vi "create odor and manifold configuration (sub-vi).vi"(7 "default directory (none)":path, 8 "error in (no error)":errorcluster, 10 "use initial config? (F)":bool, 11 "initial odor and manifold config (none)":T1) -> (0 "error out":errorcluster, 2 "operation failed?":bool, 3 "odor and manifold config out":T1)   [LabVIEW 2021]
uses:
  type-defs/odor description array (type def).ctl
  type-defs/odor info cluster (type def).ctl
  type-defs/odor selection (type def).ctl
  type-defs/odor color (type def).ctl
  type-defs/manifold configuration cluster array (type def).ctl
  type-defs/manifold configuration cluster (type def).ctl
  type-defs/manifold selection.ctl
  type-defs/single port single odor cluster.ctl
  type-defs/port number (type def).ctl
  type-defs/odor and manifold config UI states (type def).ctl
  type-defs/odor and manifold config cluster (type def).ctl
  <vilib>/Utility/error.llb/DialogType.ctl
  global-variables/global variables.vi
  <vilib>/Utility/error.llb/Error Cluster From Error Code.vi
  <vilib>/ErrorRing/Error Ring.xnode
panel:
  out "value error source":string
  in  "load config":bool
  in  "save config":bool
  in  "confirm button":bool
  out "state":T11
  out "cycle number":i32
  in  "odor config":T9 caption="Configure Odor Channels"
  in  "manifold config":T2 caption="Configure Manifold Ports"
  in  "cancel button":bool
  # "File"
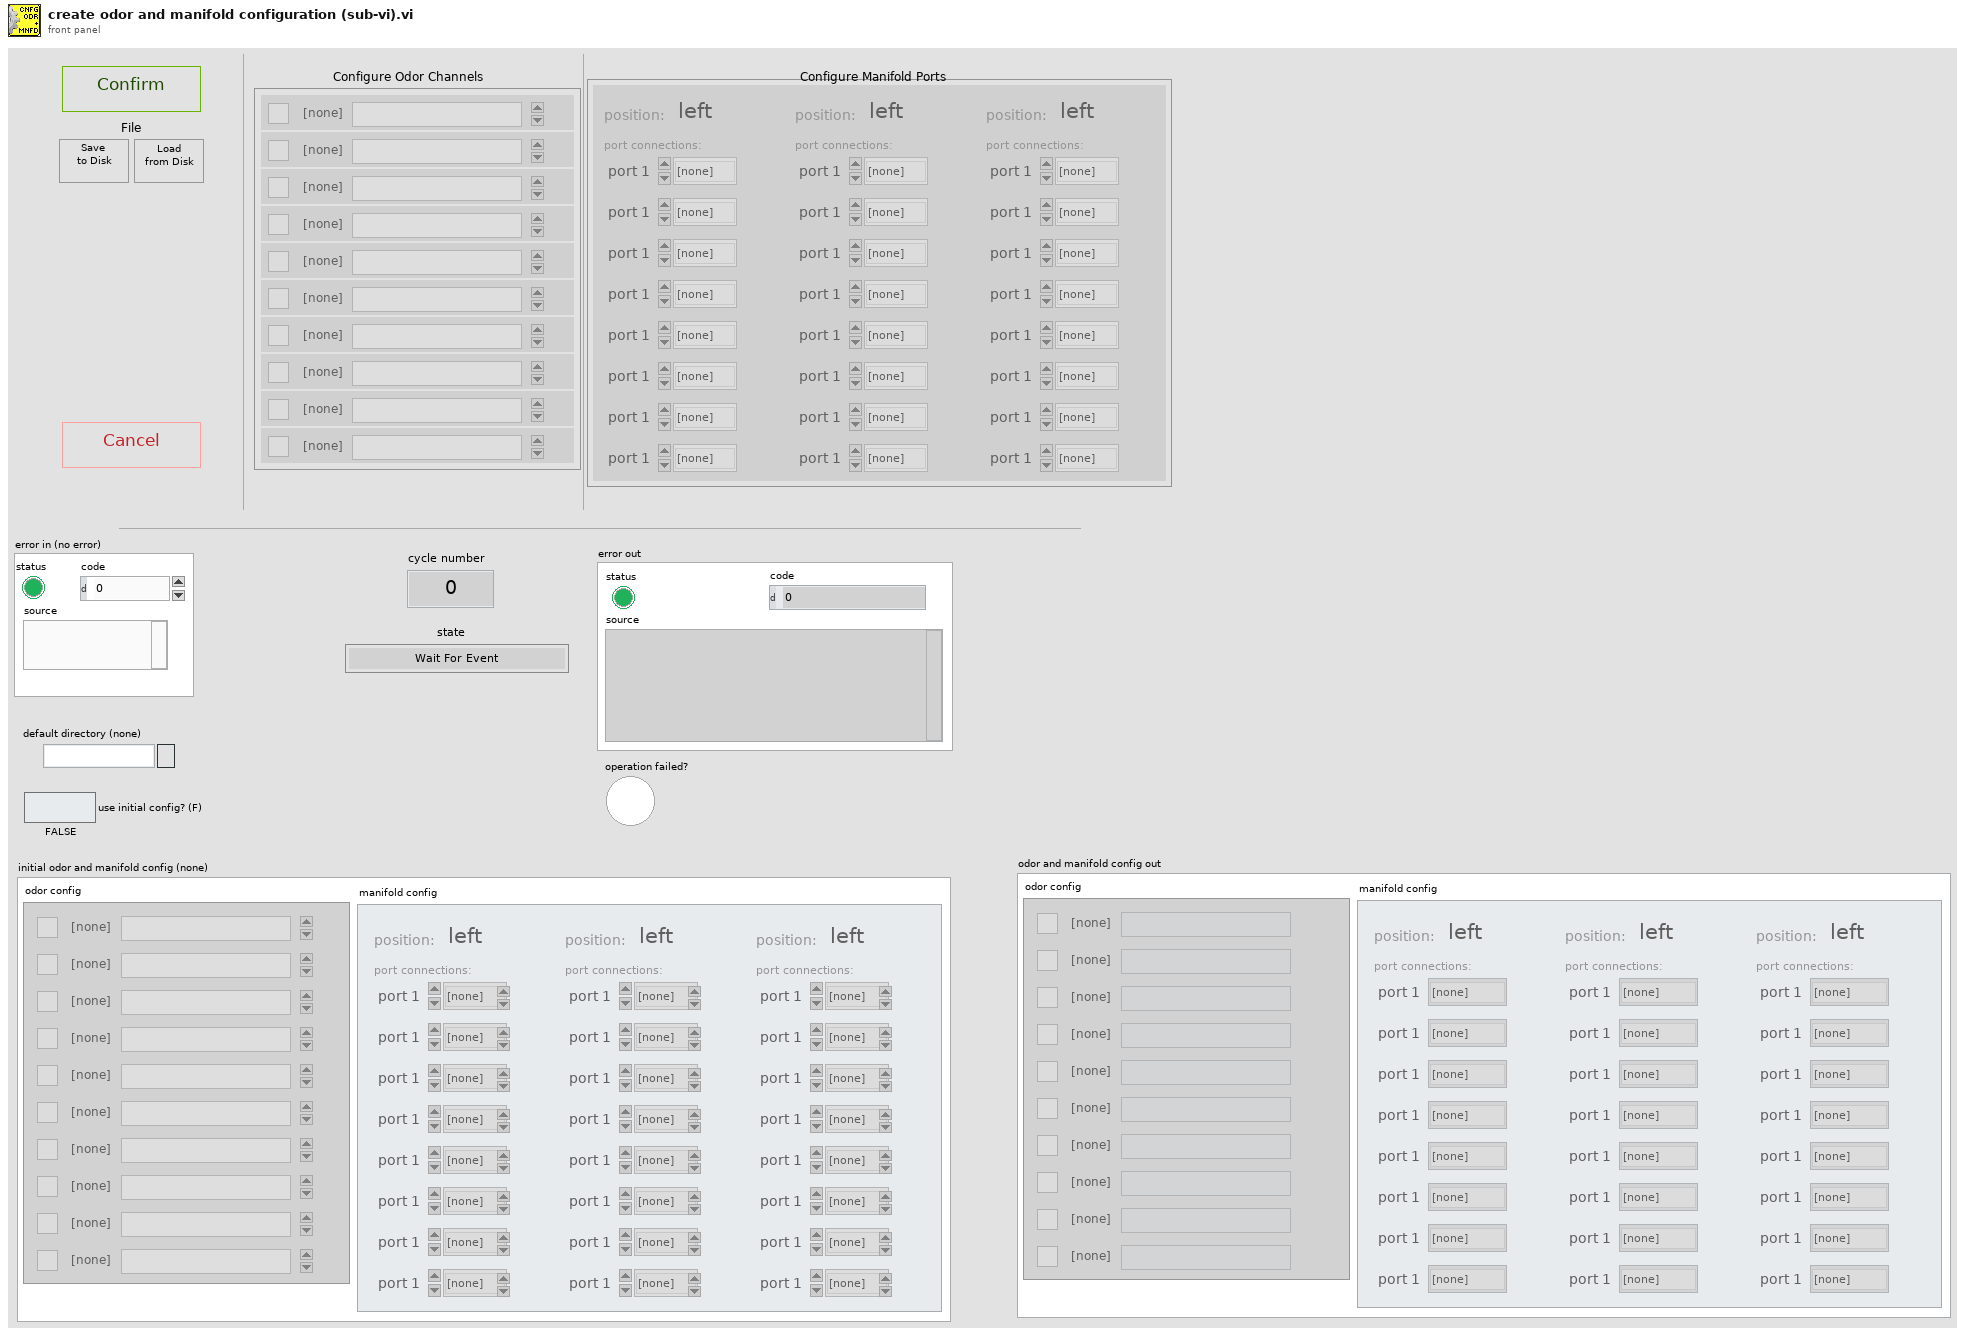
[diagram p1: front panel]
types:
  T1 = typedef "odor and manifold config cluster (type def).ctl" = cluster{"manifold config":T2, "odor config":T9}
  T2 = typedef "manifold configuration cluster array (type def).ctl" = T3[]
  T3 = typedef "manifold configuration cluster (type def).ctl" = cluster{"position:":T4, "port connections:":T5[]}
  T4 = typedef "manifold selection.ctl" = enum16{"left", "middle", "right"}
  T5 = typedef "single port single odor cluster.ctl" = cluster{"port number":T6, "connected odor":T7, "error":bool, "odor color":T8}
  T6 = typedef "port number (type def).ctl" = enum16{"port 1", "port 2", "port 3", "port 4", "port 5", "port 6", "port 7", "port 8"}
  T7 = typedef "odor selection (type def).ctl" = enum16{"[none]", "odor 1", "odor 2", "odor 3", "odor 4", "odor 5", "odor 6", "odor 7", "odor 8", "odor 9", "odor 10"}
  T8 = typedef "odor color (type def).ctl" = u16
  T9 = typedef "odor description array (type def).ctl" = T10[]
  T10 = typedef "odor info cluster (type def).ctl" = cluster{"odor channel":T7, "odor description":string, "odor color":T8, "odor channel active":bool}
  T11 = typedef "odor and manifold config UI states (type def).ctl" = enum16{"Wait For Event", "Initialize", "Update Odor Config [] Control", "Update Manifold Config [] Control", "Load Config From File", "Handle Errors", "Save Config To File", "Exit"}
  T12 = typedef "DialogType.ctl" = u16
  T13 = enum8{"Enabled", "Disabled", "Disabled and Grayed Out"}
  T14 = enum16{"open", "replace", "create", "open or create", "replace or create", "replace or create with confirmation"}
  T15 = enum16{"big-endian, network order", "native, host order", "little-endian"}
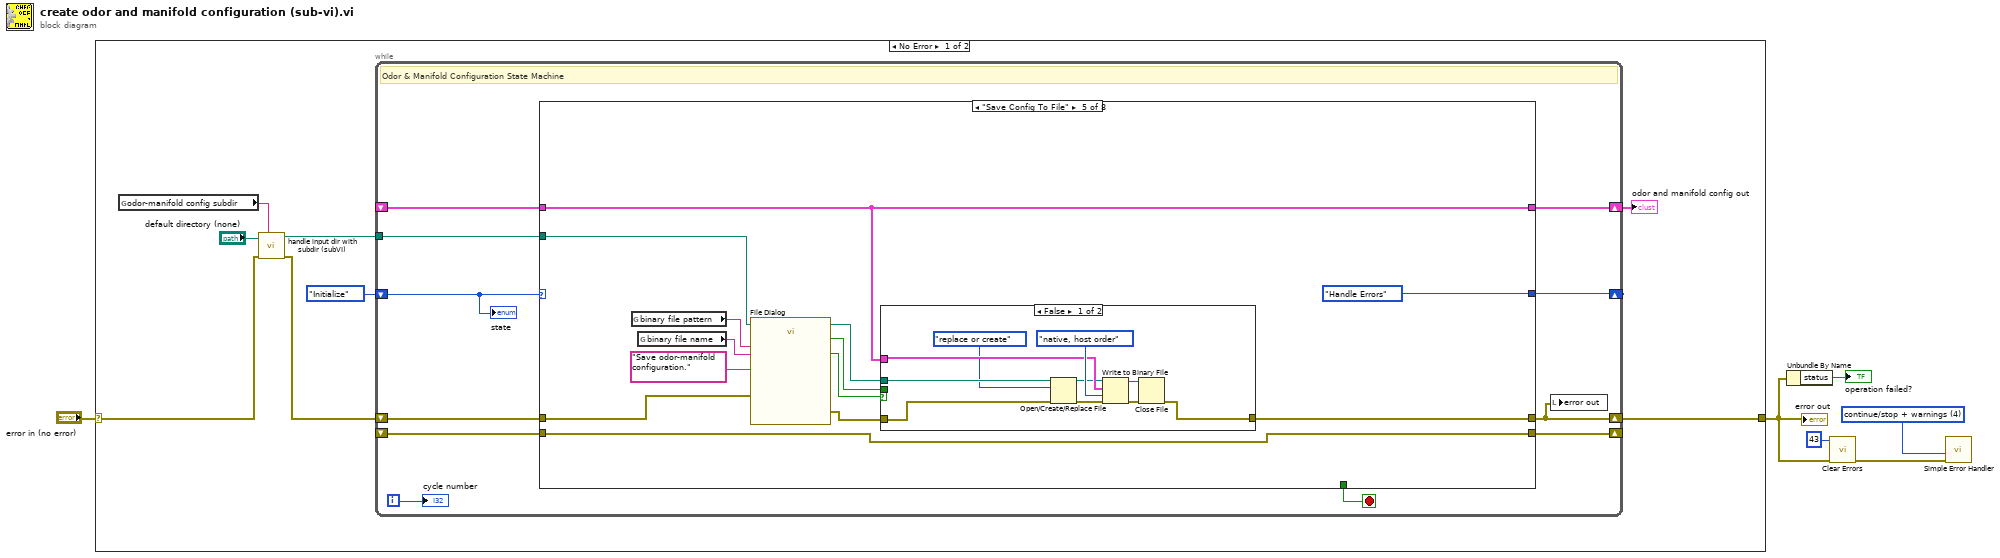
[diagram p0: block diagram]
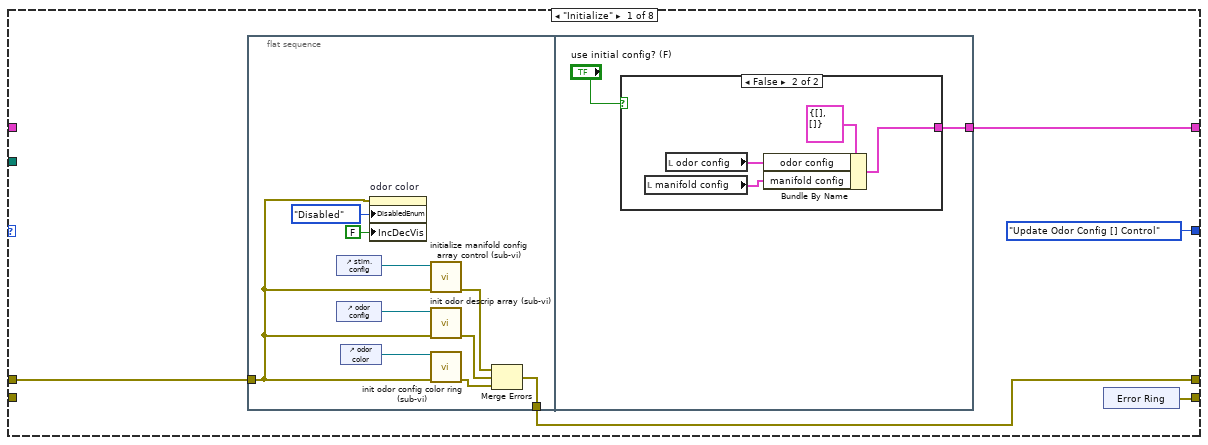
[diagram p2: hidden frame]
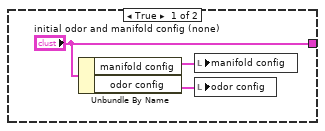
[diagram p3: hidden frame]
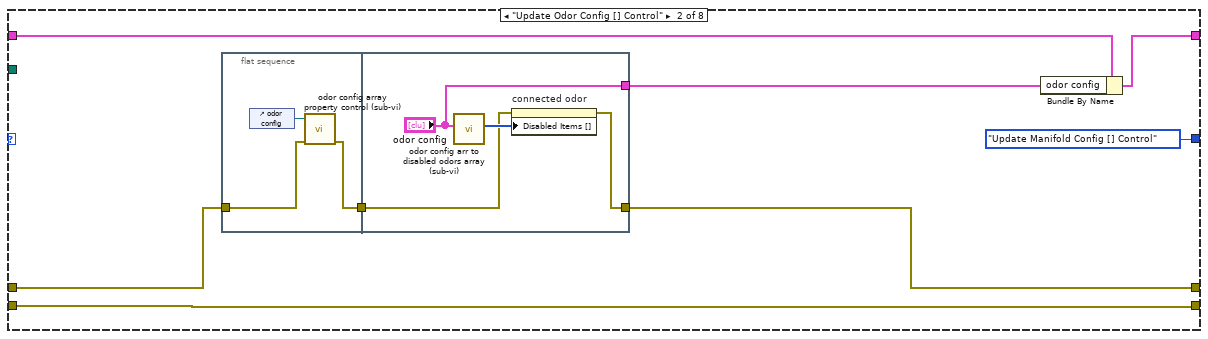
[diagram p4: hidden frame]
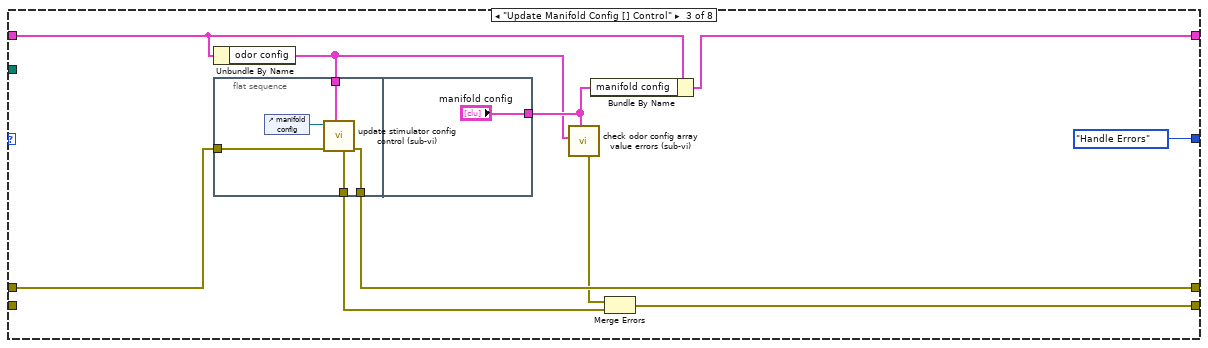
[diagram p5: hidden frame]
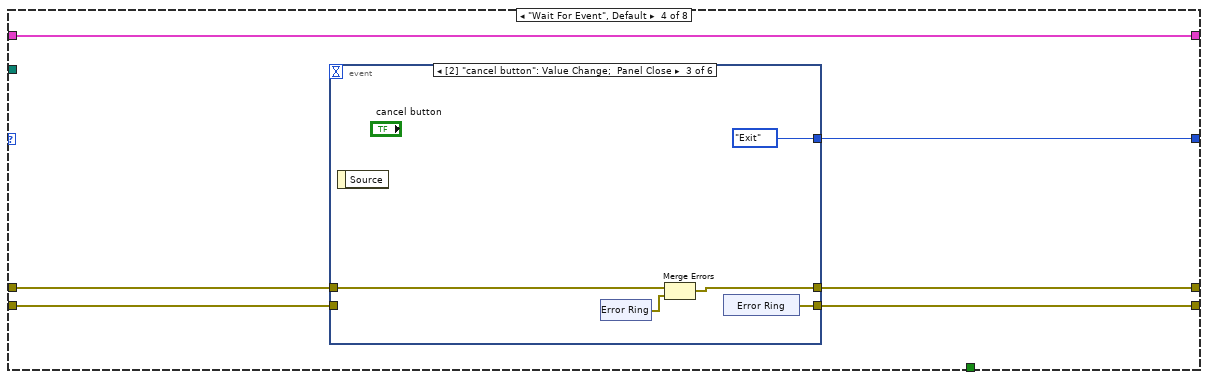
[diagram p6: hidden frame]
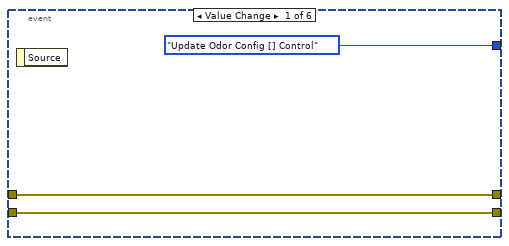
[diagram p7: hidden frame]
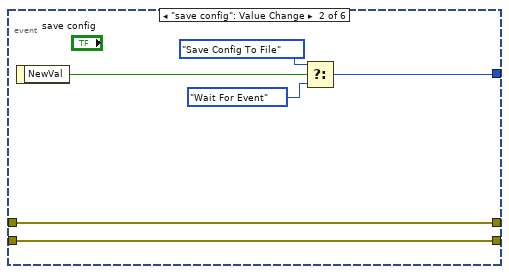
[diagram p8: hidden frame]
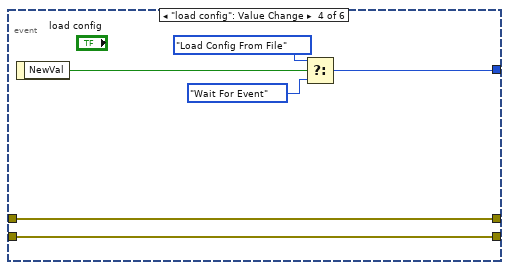
[diagram p9: hidden frame]
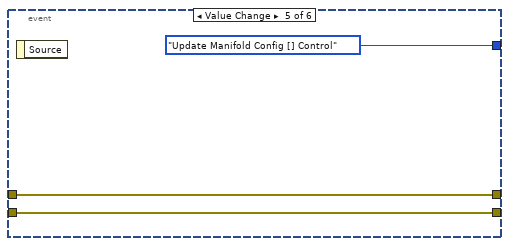
[diagram p10: hidden frame]
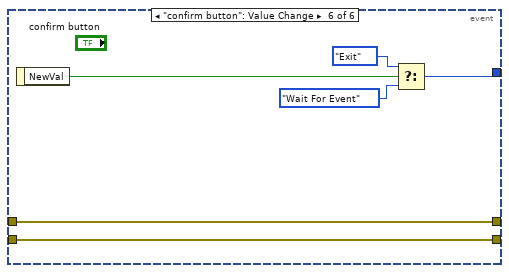
[diagram p11: hidden frame]
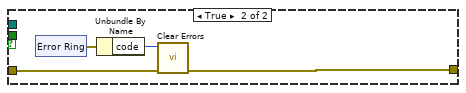
[diagram p12: hidden frame]
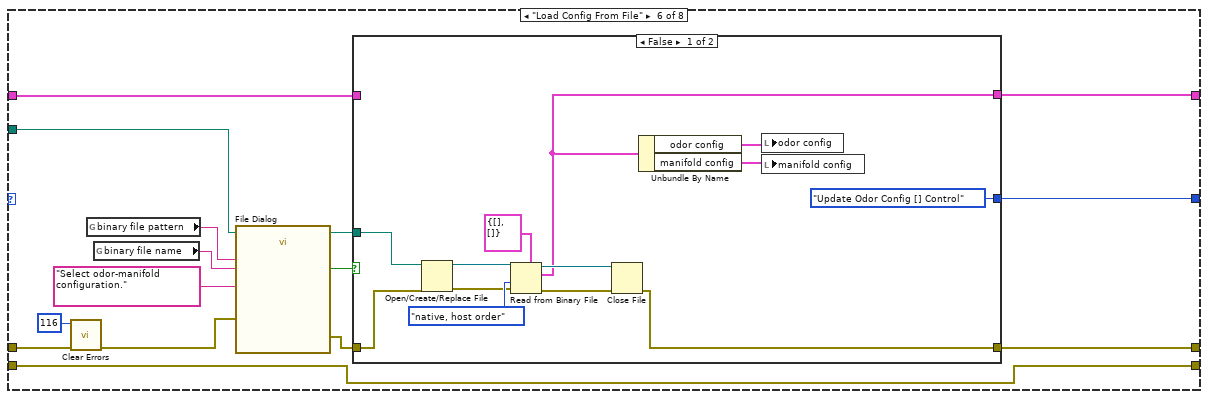
[diagram p13: hidden frame]
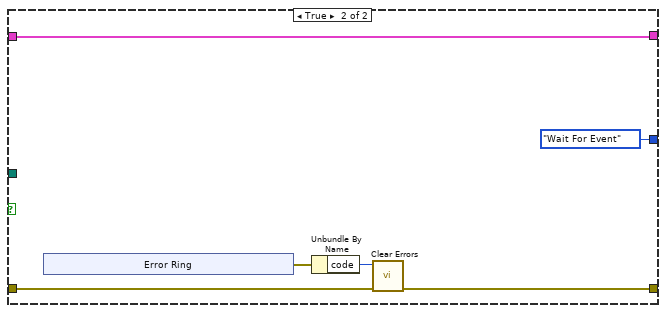
[diagram p14: hidden frame]
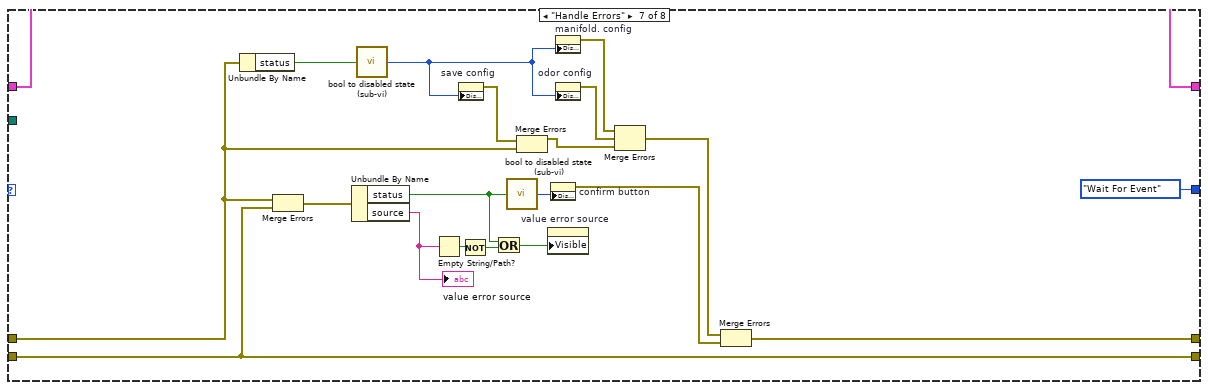
[diagram p15: hidden frame]
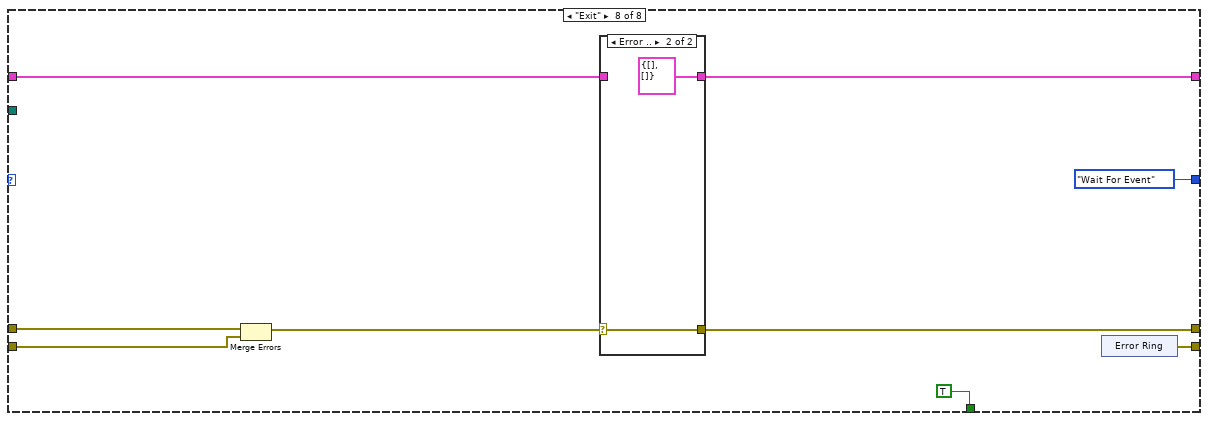
[diagram p16: hidden frame]
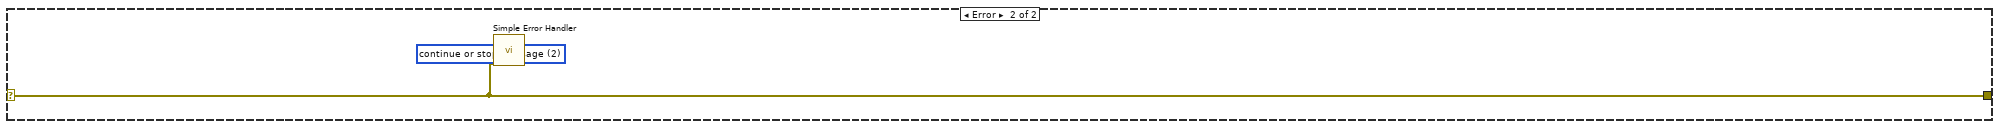
[diagram p18: hidden frame]
diagram:
  w4 = T12 4 items=["no dialog", "OK message", "continue or stop message", "OK message + warnings", "continue/stop + warnings"] ("type of dialog (OK msg:1)")
  n1 = case shown="No Error" "error in (no error)" {
    selector: "error in (no error)" -> [w10 w226]
    tunnel: [w12 w226] -> w2
    frame No Error {
      n2 = global read "global variables.vi" "odor-manifold config subdir"() -> (w7:string)
      n3 = call "handle input dir with subdir (subVI).vi"("subdir name (none)"=w7, "error in (no error)"=w10, "starting directory (none)"="default directory (none)") -> ("error out"=w9:errorcluster, "dirctory path"=w11:path)  [unwired: 7 in]
      n4 = while {
        shift-right: [w20] -> w12
        shift-left: w9 -> [w25]
        shift-right: [w22] -> _
        shift-left: odor_and_manifold_config_UI_states_(type_def)."Initialize" ("Enum") -> [w21]
        shift-right: [w19] -> w13
        shift-left: _ -> [w18]
        shift-right: [w17] -> _
        shift-left: _ -> [w16]
        tunnel: w11 -> [w15]
        i -> [w23]
        stop <- w24 stop-if-true
        # "Odor & Manifold Configuration State Machine"
        n5 = case shown="\"Save Config To File\"" w21 {
          tunnel: w25 -> [w30 w57 w75 w85 w128 w160 w196 w214]
          tunnel: [w26 w56 w71 w84 w134 w166 w200 w217] -> w20
          tunnel: [odor_and_manifold_config_UI_states_(type_def)."Update Odor Config [] Control" ("Enum") odor_and_manifold_config_UI_states_(type_def)."Update Manifold Config [] Control" ("Enum") odor_and_manifold_config_UI_states_(type_def)."Handle Errors" ("Enum") w87 odor_and_manifold_config_UI_states_(type_def)."Handle Errors" ("Enum") w165 odor_and_manifold_config_UI_states_(type_def)."Wait For Event" ("Enum") odor_and_manifold_config_UI_states_(type_def)."Wait For Event" ("Enum")] -> w22
          tunnel: [_ _ _ _ _ _ _ TRUE] -> w24
          tunnel: [w28 w52 w73 w86 w132 w164 w205 w216] -> w19
          tunnel: w18 -> [_ w54 w70 w86 w132 w158 w205 w215]
          tunnel: [w27 w51 w72 w82 w131 w163 w202 w211] -> w17
          tunnel: w16 -> [_ w51 _ w83 w131 w163 w202 w212]
          tunnel: w15 -> [_ _ _ _ w123 w155 _ _]
          frame "Initialize" {
            n6 = flat-sequence {
              tunnel: w30 -> [w32]
              tunnel: [w35] -> w26
              tunnel: [w42] -> w28
              frame #0 {
                n7 = control-ref of="stim. config"() -> (w38:refnum<vi>)
                n8 = control-ref of="odor config"() -> (w37:refnum<vi>)
                n9 = control-ref of="odor color"() -> (w36:refnum<vi>)
                n10 = property on="odor color" class="Ring (strict)"(error in=w32, "DisabledEnum"=T13."Disabled" ("Disabled"), "IncDecVis"=FALSE ("Increment/Decrement Visible?")) -> ()  [unwired: 1 in, 2 out]
                n11 = call "initialize manifold config array control (sub-vi).vi"("error in (no error)"=w32, "stimulator config array refnum"=w38) -> ("error out"=w41:errorcluster)  [unwired: 8 in, 1 out]
                n12 = call "init odor descrip array (sub-vi).vi"("error in (no error)"=w32, "array refnum"=w37) -> ("error out"=w40:errorcluster)  [unwired: 8 in, 1 out]
                n13 = call "init odor config color ring (sub-vi).vi"("error in (no error)"=w32, "ring refnum"=w36) -> ("error out"=w39:errorcluster)  [unwired: 8 in, 1 out]
                n14 = Merge Errors(w41, w40, w39) -> (w35:errorcluster)
              }
              frame #1 {
                n15 = case shown="False" "use initial config? (F)" {
                  tunnel: ["initial odor and manifold config (none)" w47] -> w42
                  frame True {
                    n16 = Unbundle By Name("initial odor and manifold config (none)") -> ("manifold config"=w44:T2, "odor config"=w45:T9)
                    n17 = local write "manifold config"(w44) -> ()
                    n18 = local write "odor config"(w45) -> ()
                  }
                  frame False {
                    n19 = local read "manifold config"() -> (w48:T2)
                    n20 = local read "odor config"() -> (w49:T9)
                    n21 = Bundle By Name(cluster=T1 {"manifold config"=[], "odor config"=[]} ("Cluster"), "odor config"=w49, "manifold config"=w48) -> (w47:T1)
                  }
                }
              }
            }
            n22 = xnode "Error Ring"() -> ("error out"=w27:errorcluster)
          }
          frame "Update Odor Config [] Control" {
            n23 = flat-sequence {
              tunnel: [w61] -> w58
              tunnel: w57 -> [w60]
              tunnel: w58 -> [w64]
              tunnel: [w63] -> w56
              tunnel: ["odor config"] -> w53
              frame #0 {
                n24 = control-ref of="odor config"() -> (w59:refnum<vi>)
                n25 = call "odor config array property control (sub-vi).vi"("error in (no error)"=w60, "odor config array refnum"=w59) -> ("error out"=w61:errorcluster)  [unwired: 8 in, 1 out]
              }
              frame #1 {
                n26 = call "odor config arr to disabled odors array (sub-vi).vi"("odor descriptions"="odor config") -> ("Disabled Items []"=w65:i32[])  [unwired: 10 in]
                n27 = property on="connected odor" class="Enum (strict)"(error in=w64, "Disabled Items []"=w65) -> (error out=w63:errorcluster)  [unwired: 1 in, 1 out]
              }
            }
            n28 = Bundle By Name(cluster=w54, "odor config"=w53) -> (w52:T1)
          }
          frame "Update Manifold Config [] Control" {
            n29 = Unbundle By Name(w70) -> ("odor config"=w66:T9)
            n30 = flat-sequence {
              tunnel: w75 -> [w79]
              tunnel: [w78] -> w69
              tunnel: [w77] -> w71
              tunnel: w66 -> [w76]
              tunnel: ["manifold config"] -> w67
              frame #0 {
                n31 = control-ref of="manifold config"() -> (w80:refnum<vi>)
                n32 = call "update stimulator config control (sub-vi).vi"("odor config array"=w76, "error in (no error)"=w79, "manifold config array refnum"=w80) -> ("error out"=w77:errorcluster, "value error out"=w78:errorcluster)  [unwired: 6 in, 1 out]
              }
              frame #1 {
              }
            }
            n33 = call "check odor config array value errors (sub-vi).vi"("manifold configuration array"=w67, "odor config array"=w66) -> ("value error"=w68:errorcluster)  [unwired: 9 in]
            n34 = Bundle By Name(cluster=w70, "manifold config"=w67) -> (w73:T1)
            n35 = Merge Errors(w68, w69) -> (w72:errorcluster)
          }
          frame "Wait For Event", Default {
            n36 = event shown="[2] \"cancel button\": Value Change;  Panel Close" {
              selector: _ -> [_ _ _ _ _ _]
              dyn-events: _ -> [_ _ _ _ _ _]
              timeout: _ -> [_ _ _ _ _ _]
              tunnel: [odor_and_manifold_config_UI_states_(type_def)."Update Odor Config [] Control" ("Enum") w93 odor_and_manifold_config_UI_states_(type_def)."Exit" ("Enum") w109 odor_and_manifold_config_UI_states_(type_def)."Update Manifold Config [] Control" ("Enum") w119] -> w87
              tunnel: w85 -> [w89 w92 w99 w108 w114 w117]
              tunnel: [w89 w92 w97 w108 w114 w117] -> w84
              tunnel: w83 -> [w88 w91 _ w107 w113 w116]
              tunnel: [w88 w91 w100 w107 w113 w116] -> w82
              event Value Change {
                n37 = event-data() -> ()  [unwired: 1 in, 1 out]
              }
              event "save config": Value Change {
                n38 = event-data() -> ("NewVal"=w96:bool)  [unwired: 1 in]
                n39 = Select(t=odor_and_manifold_config_UI_states_(type_def)."Save Config To File", s=w96, f=odor_and_manifold_config_UI_states_(type_def)."Wait For Event" ("Enum")) -> (s? t:f=w93:T11)
              }
              event "cancel button": Value Change; Panel Close {
                n40 = event-data() -> ()  [unwired: 1 in, 1 out]
                n41 = xnode "Error Ring"() -> ("error out"=w98:errorcluster)
                n42 = Merge Errors(w99, w98) -> (w97:errorcluster)
                n43 = xnode "Error Ring"() -> ("error out"=w100:errorcluster)
              }
              event "load config": Value Change {
                n44 = event-data() -> ("NewVal"=w112:bool)  [unwired: 1 in]
                n45 = Select(t=odor_and_manifold_config_UI_states_(type_def)."Load Config From File", s=w112, f=odor_and_manifold_config_UI_states_(type_def)."Wait For Event" ("Enum")) -> (s? t:f=w109:T11)
              }
              event Value Change {
                n46 = event-data() -> ()  [unwired: 1 in, 1 out]
              }
              event "confirm button": Value Change {
                n47 = event-data() -> ("NewVal"=w121:bool)  [unwired: 1 in]
                n48 = Select(t=odor_and_manifold_config_UI_states_(type_def)."Exit", s=w121, f=odor_and_manifold_config_UI_states_(type_def)."Wait For Event" ("Enum")) -> (s? t:f=w119:T11)
              }
            }
          }
          frame "Save Config To File" {
            n49 = global read "global variables.vi" "binary file pattern"() -> (w124:string)
            n50 = global read "global variables.vi" "binary file name"() -> (w125:string)
            n51 = call "File Dialog"("start path"=w123, "prompt"="Save odor-manifold configuration.", "error in"=w128, "pattern (all files)"=w124, "pattern label"=w125) -> ("selected path"=w129:path, "exists"=w122:bool, "cancelled"=w130:bool, "error out"=w127:errorcluster)  [unwired: 7 in]
            n52 = case shown="False" w130 {
              tunnel: [w141 w146] -> w134
              tunnel: w132 -> [w140 _]
              tunnel: w127 -> [w139 w145]
              tunnel: w129 -> [w136 _]
              tunnel: w122 -> [_ _]
              frame False {
                n53 = Open/Create/Replace File(file path (use dialog)=w136, error in=w139, operation (0:open)=T14."replace or create") -> (refnum out=w137:refnum<file>, error out=w138:errorcluster)  [unwired: 3 in, 1 out]
                n54 = Write to Binary File(file (use dialog)=w137, data=w140, error in=w138, 9:T15."native, host order" ("byte order (0:big-endian, network order)")) -> (refnum out=w143:refnum<file>, error out=w144:errorcluster)  [unwired: 2 in, 1 out]
                n55 = Close File(refnum=w143, error in=w144) -> (error out=w141:errorcluster)  [unwired: 1 out]
              }
              frame True {
                n56 = xnode "Error Ring"() -> ("error out"=w148:errorcluster)
                n57 = Unbundle By Name(w148) -> ("code"=w147:i32)
                n58 = call <vilib>:"Clear Errors.vi"("error in (no error)"=w145, "specific error code to clear (0: all)"=w147) -> ("error out"=w146:errorcluster)  [unwired: 4 in, 1 out]
              }
            }
          }
          frame "Load Config From File" {
            n59 = call <vilib>:"Clear Errors.vi"("error in (no error)"=w160, "specific error code to clear (0: all)"=116) -> ("error out"=w154:errorcluster)  [unwired: 4 in, 1 out]
            n60 = global read "global variables.vi" "binary file pattern"() -> (w157:string)
            n61 = global read "global variables.vi" "binary file name"() -> (w156:string)
            n62 = call "File Dialog"("start path"=w155, "prompt"="Select odor-manifold configuration.", "error in"=w154, "pattern (all files)"=w157, "pattern label"=w156) -> ("selected path"=w167:path, "cancelled"=w161:bool, "error out"=w162:errorcluster)  [unwired: 7 in, 1 out]
            n63 = case shown="False" w161 {
              tunnel: w162 -> [w170 w185]
              tunnel: w167 -> [w171 _]
              tunnel: [w174 w184] -> w166
              tunnel: [odor_and_manifold_config_UI_states_(type_def)."Update Odor Config [] Control" ("Enum") odor_and_manifold_config_UI_states_(type_def)."Wait For Event" ("Enum")] -> w165
              tunnel: w158 -> [_ w181]
              tunnel: [w175 w181] -> w164
              frame False {
                n64 = Open/Create/Replace File(file path (use dialog)=w171, error in=w170) -> (refnum out=w168:refnum<file>, error out=w169:errorcluster)  [unwired: 4 in, 1 out]
                n65 = Read from Binary File(5:T1 {"manifold config"=[], "odor config"=[]} ("Cluster"), 8:w169, 9:T15."native, host order" ("byte order (0:big-endian, network order)"), 11:w168) -> (0:w180:errorcluster, 2:w175:T1, 3:w179:refnum<file>)  [unwired: 2 in, 1 out]
                n66 = Close File(refnum=w179, error in=w180) -> (error out=w174:errorcluster)  [unwired: 1 out]
                n67 = Unbundle By Name(w175) -> ("odor config"=w172:T9, "manifold config"=w173:T2)
                n68 = local write "odor config"(w172) -> ()
                n69 = local write "manifold config"(w173) -> ()
              }
              frame True {
                n70 = xnode "Error Ring"() -> ("error out"=w183:errorcluster)
                n71 = Unbundle By Name(w183) -> ("code"=w182:i32)
                n72 = call <vilib>:"Clear Errors.vi"("error in (no error)"=w185, "specific error code to clear (0: all)"=w182) -> ("error out"=w184:errorcluster)  [unwired: 4 in, 1 out]
              }
            }
          }
          frame "Handle Errors" {
            n73 = Unbundle By Name(w196) -> ("status"=w198:bool)
            n74 = Merge Errors(w196, w202) -> (w197:errorcluster)
            n75 = Unbundle By Name(w197) -> ("status"=w194:bool, "source"=w192:string)
            "value error source" <- w192
            n76 = call "bool to disabled state (sub-vi).vi"("error?"=w198) -> ("disabled"=w203:T13)
            n77 = Empty String/Path?(string/path=w192) -> (empty?=w193:bool)
            n78 = property on="save config" class="Bool"("DisabledEnum"=w203) -> (error out=w210:errorcluster)  [unwired: 2 in, 1 out]
            n79 = Not(x=w193) -> (.not. x?=w191:bool)
            n80 = Or(x=w194, y=w191) -> (x .or. y?=w195:bool)
            n81 = call "bool to disabled state (sub-vi).vi"("error?"=w194) -> ("disabled"=w201:T13)
            n82 = Merge Errors(w210, w196) -> (w209:errorcluster)
            n83 = property on="value error source" class="Str"("Visible"=w195) -> ()  [unwired: 2 in, 2 out]
            n84 = property on="confirm button" class="Bool"("DisabledEnum"=w201) -> (error out=w199:errorcluster)  [unwired: 2 in, 1 out]
            n85 = property on="manifold. config" class="Arr (strict)"("DisabledEnum"=w203) -> (error out=w206:errorcluster)  [unwired: 2 in, 1 out]
            n86 = property on="odor config" class="Arr (strict)"("DisabledEnum"=w203) -> (error out=w207:errorcluster)  [unwired: 2 in, 1 out]
            n87 = Merge Errors(w206, w207, w209) -> (w204:errorcluster)
            n88 = Merge Errors(w204, w199) -> (w200:errorcluster)
          }
          frame "Exit" {
            n89 = Merge Errors(w214, w212) -> (w213:errorcluster)
            n90 = case shown="Error .." w213 {
              selector: w213 -> [w222 w223]
              tunnel: [w222 w223] -> w217
              tunnel: [w221 T1 {"manifold config"=[], "odor config"=[]} ("Cluster")] -> w216
              tunnel: w215 -> [w221 _]
              frame No Error {
              }
              frame Error {
              }
            }
            n91 = xnode "Error Ring"() -> ("error out"=w211:errorcluster)
          }
        }
        n92 = local write "error out"(w20) -> ()
        "state" <- w21
        "cycle number" <- w23
      }
      "odor and manifold config out" <- w13
    }
    frame Error {
      w225 = T12 2 items=["no dialog", "OK message", "continue or stop message", "OK message + warnings", "continue/stop + warnings"] ("type of dialog (OK msg:1)")
      n93 = call <vilib>:"Simple Error Handler.vi"("type of dialog (OK msg:1)"=w225, "error in (no error)"=w226) -> ()  [unwired: 3 in, 5 out]
    }
  }
  "error out" <- w2
  n94 = Unbundle By Name(w2) -> ("status"=→"operation failed?":bool)
  n95 = call <vilib>:"Clear Errors.vi"("error in (no error)"=w2, "specific error code to clear (0: all)"=43) -> ("error out"=w5:errorcluster)  [unwired: 4 in, 1 out]
  n96 = call <vilib>:"Simple Error Handler.vi"("type of dialog (OK msg:1)"=w4, "error in (no error)"=w5) -> ()  [unwired: 3 in, 5 out]
